vi "Data(dictionary) to XY.vi"(6 "dimension size (hmm)":i32=400, 7 "chopper params":T1, 8 "error in (no error)":errorcluster, 9 "IV Y wavename":string, 10 "IV X wavename":string, 11 "Data (Dictionary)":T2[](array[typedef])) -> (0 "error out":errorcluster, 3 "wacky arary":cluster{dbl[], dbl[]}[](array[cluster]))   [LabVIEW 2016]
uses:
  <userlib>/LevyLab/LV to ITX/Data/Typedefs/Dictionary--cluster.ctl
  ctl/Chopper Parameters -- Cluster.ctl
  <userlib>/LevyLab/LV to ITX/Data/Data.lvclass
panel:
  out "x/y":dbl
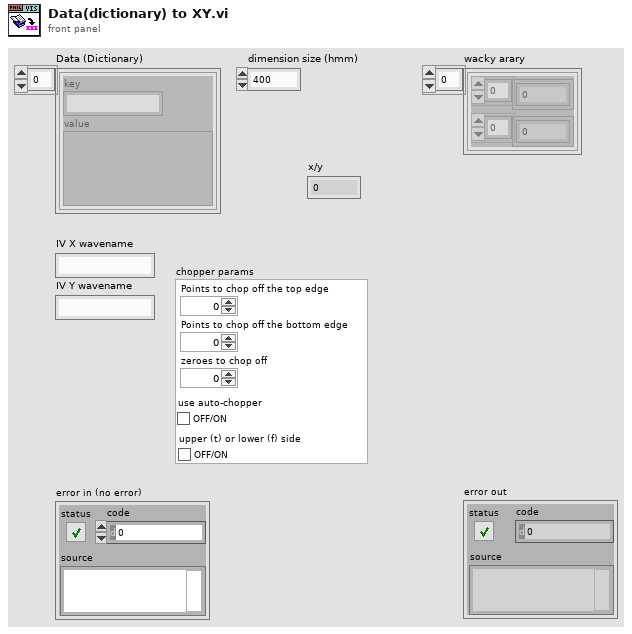
[diagram p1: front panel]
types:
  T1 = typedef "Chopper Parameters -- Cluster.ctl" = cluster{"Points to chop off the top edge":i32, "Points to chop off the bottom edge":i32, "zeroes to chop off":i32, "use auto-chopper":bool, "upper (t) or lower (f) side":bool}
  T2 = typedef "Data.lvclass/Dictionary--cluster.ctl" = cluster{"key":string, "value":variant}
  T3 = typedef "Dictionary Object RefNum__ogtk.ctl" = refnum<k1>
  T4 = cluster{"x arr possibly chopped":dbl[], "y arr possibly chopped":dbl[]}
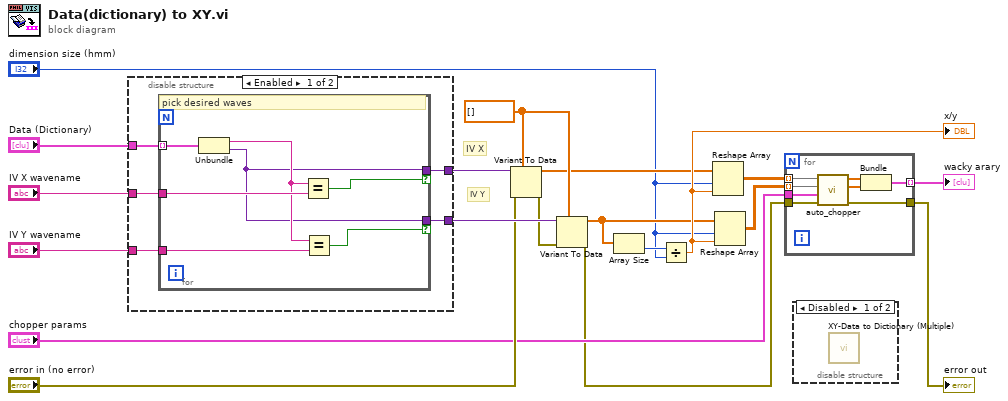
[diagram p0: block diagram]
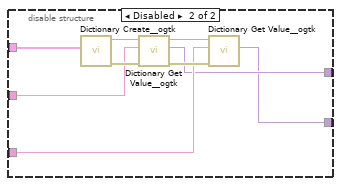
[diagram p2: hidden frame]
diagram:
  w15 = dbl[] []
  # "IV Y"
  # "IV X"
  n1 = disable-structure shown="Enabled" {
    disable-tunnel: [w24 w33] -> w19
    disable-tunnel: [w23 w32] -> w18
    disable-tunnel: "Data (Dictionary)" -> [w22 w36]
    disable-tunnel: "IV X wavename" -> [w21 w35]
    disable-tunnel: "IV Y wavename" -> [w20 w34]
    frame Enabled {
      n2 = for {
        tunnel: w22 -> [w31] mode=indexing
        tunnel: w21 -> [w30]
        tunnel: w20 -> [w28]
        tunnel: [w27] -> w24 if=w26
        tunnel: [w27] -> w23 if=w25
        # "pick desired waves"
        n3 = Unbundle(w31) -> ("key"=w29:string, "value"=w27:variant)
        n4 = Equal?(x=w29, y=w30) -> (x = y?=w26:bool)
        n5 = Equal?(x=w29, y=w28) -> (x = y?=w25:bool)
      }
    }
    frame Disabled {
      n6 = call <userlib>:"Dictionary Create__ogtk.vi"("initial dictionary (empty)"=w36) -> ("error out"=w37:errorcluster, "dictionary out"=w38:T3)  [unwired: 9 in]
      n7 = call <userlib>:"Dictionary Get Value__ogtk.vi"("error in"=w37, "key"=w35, "dictionary"=w38) -> ("error out"=w40:errorcluster, "value"=w33:variant, "dictionary out"=w39:T3)  [unwired: 5 in, 1 out]
      n8 = call <userlib>:"Dictionary Get Value__ogtk.vi"("error in"=w40, "key"=w34, "dictionary"=w39) -> ("value"=w32:variant)  [unwired: 5 in, 3 out]
    }
  }
  n9 = Variant To Data(error in="error in (no error)", type=w15, Variant=w19) -> (data=w8:dbl[], error out=w17:errorcluster)
  n10 = Variant To Data(error in=w17, type=w15, Variant=w18) -> (data=w9:dbl[], error out=w6:errorcluster)
  n11 = Array Size(array=w9) -> (size(s)=w11:i32)
  n12 = Divide(x=w11, y="dimension size (hmm)") -> (x/y=w10:dbl)
  "x/y" <- w10
  n13 = Reshape Array(w8, "dimension size (hmm)", w10) -> (w14:dbl[][])
  n14 = Reshape Array(w9, "dimension size (hmm)", w10) -> (w13:dbl[][])
  n15 = for {
    tunnel: w14 -> [w46] mode=indexing
    tunnel: w13 -> [w45] mode=indexing
    tunnel: [w48] -> w12 mode=indexing
    tunnel: "chopper params" -> [w47]
    tunnel: w6 -> [w42]
    tunnel: [w41] -> w2
    n16 = call "auto_chopper.vi"("error in (no error)"=w42, "chopper params"=w47, "y arr"=w45, "x arr"=w46) -> ("error out"=w41:errorcluster, "y arr possibly chopped"=w43:dbl[], "x arr possibly chopped"=w44:dbl[])  [unwired: 1 in, 4 out]
    n17 = Bundle("x arr possibly chopped"=w44, "y arr possibly chopped"=w43) -> (w48:T4)  [unwired: 1 in]
  }
  "error out" <- w2
  "wacky arary" <- w12
  n18 = disable-structure shown="Disabled" {
    frame Disabled {
      n19 = call <userlib>:"XY-Data to Dictionary (Multiple).vi"() -> ()  [unwired: 10 in, 2 out]
    }
    frame Enabled {
    }
  }
